vi "set file meta.vi"(8 "error in (no error)":errorcluster, 11 "pulse_gen_and_detect_p2p in":refnum<class "pulse_gen_and_detect_p2p.lvclass">) -> (0 "error out":errorcluster, 3 "pulse_gen_and_detect_p2p out":refnum<class "pulse_gen_and_detect_p2p.lvclass">)   [LabVIEW 2021, in "pulse_gen_and_detect_p2p.lvclass"]
uses:
  pulse_gen_and_detect_p2p.lvclass
  pulse_gen_and_detect_p2p.lvclass/pulse_gen_and_detect_p2p.ctl
  pulse_tx_vis/CTL/device_mode.ctl
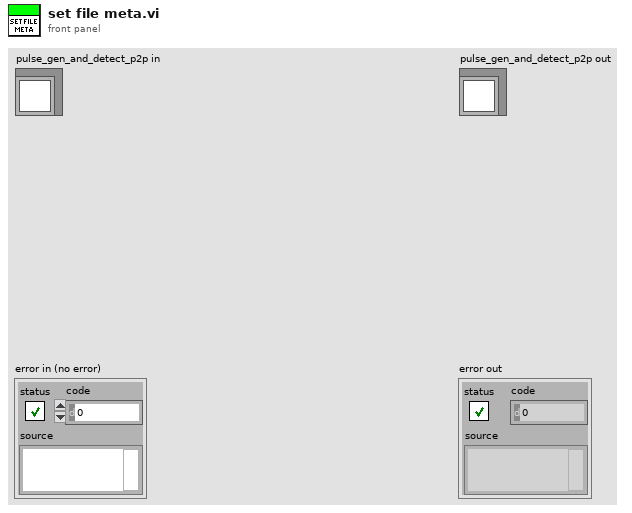
[diagram p1: front panel]
types:
  T1 = typedef "device_mode.ctl" = enum16{"USRP - 180MHz", "5785 - 2*180MHz", "5785 - 3.2GHz", "P2P - VST", "5785 2*1.6GHz", "P2P Tx and Rx"}
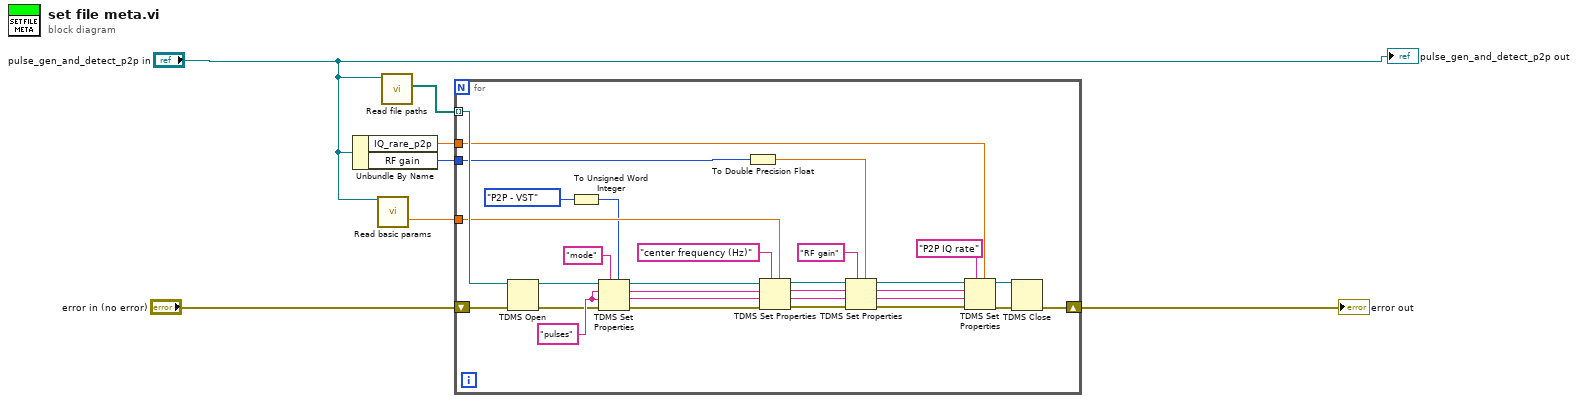
[diagram p0: block diagram]
diagram:
  n1 = Unbundle By Name("pulse_gen_and_detect_p2p in") -> ("IQ_rare_p2p"=w4:dbl, "RF gain"=w5:i32)
  n2 = call-dynamic "Read basic params.vi"("device_type in"="pulse_gen_and_detect_p2p in") -> ("center frequency (Hz)"=w6:dbl)  [unwired: 13 in, 5 out]
  n3 = call-dynamic "Read file paths.vi"("device_type in"="pulse_gen_and_detect_p2p in") -> ("file paths"=w7:path[])  [unwired: 8 in, 2 out]
  n4 = for {
    tunnel: w7 -> [w35] mode=indexing
    shift-right: [w25] -> w1
    shift-left: "error in (no error)" -> [w26]
    tunnel: w6 -> [w27]
    tunnel: w5 -> [w9]
    tunnel: w4 -> [w14]
    w37 = "pulses" ("channel name")
    n5 = TDMS Open(8:w26, 11:w35) -> (0:w34:errorcluster, 3:w36:refnum<k34>)  [unwired: 5 in]
    n6 = To Unsigned Word Integer(number=device_mode."P2P - VST" ("Mode")) -> (unsigned 16bit integer=w10:u16)
    n7 = TDMS Set Properties(5:w10, 7:"mode", 8:w34, 9:w37, 10:w37, 11:w36) -> (0:w31:errorcluster, 1:w30:string, 2:w29:string, 3:w32:refnum<k34>)
    n8 = To Double Precision Float(number=w9) -> (double precision float=w8:dbl)
    n9 = TDMS Set Properties(5:w27, 7:"center frequency (Hz)", 8:w31, 9:w30, 10:w29, 11:w32) -> (0:w20:errorcluster, 1:w21:string, 2:w22:string, 3:w23:refnum<k34>)
    n10 = TDMS Set Properties(5:w8, 7:"RF gain", 8:w20, 9:w21, 10:w22, 11:w23) -> (0:w15:errorcluster, 1:w16:string, 2:w17:string, 3:w18:refnum<k34>)
    n11 = TDMS Set Properties(5:w14, 7:"P2P IQ rate", 8:w15, 9:w16, 10:w17, 11:w18) -> (0:w12:errorcluster, 3:w13:refnum<k34>)  [unwired: 2 out]
    n12 = TDMS Close(8:w12, 11:w13) -> (0:w25:errorcluster)  [unwired: 1 out]
  }
  "error out" <- w1
  "pulse_gen_and_detect_p2p out" <- "pulse_gen_and_detect_p2p in"
